vi "4155C Split array.vi"(0 "Number of VAR2 steps":i32, 1 "Y2 data in":dbl[](array[numeric]) format="%.2f", 2 "X data in":dbl[](array[numeric]) format="%.2f", 3 "Y1 data in":dbl[](array[numeric]) format="%.2f", 4 "Y3 data in":dbl[](array[numeric]) format="%.2f", 5 "error in (no error)":errorcluster, 8 "Absolute val?":bool=TRUE) -> (6 "Array of clusters":cluster{"Y data in":dbl[], "X data in":dbl[]}[](array[cluster]) {"X data in" format="%.2f"; "Y data in" format="%.2f"}, 7 "error out":errorcluster)   [LabVIEW 2019]
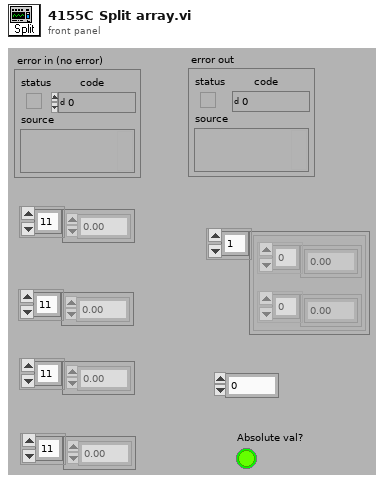
[diagram p1: front panel]
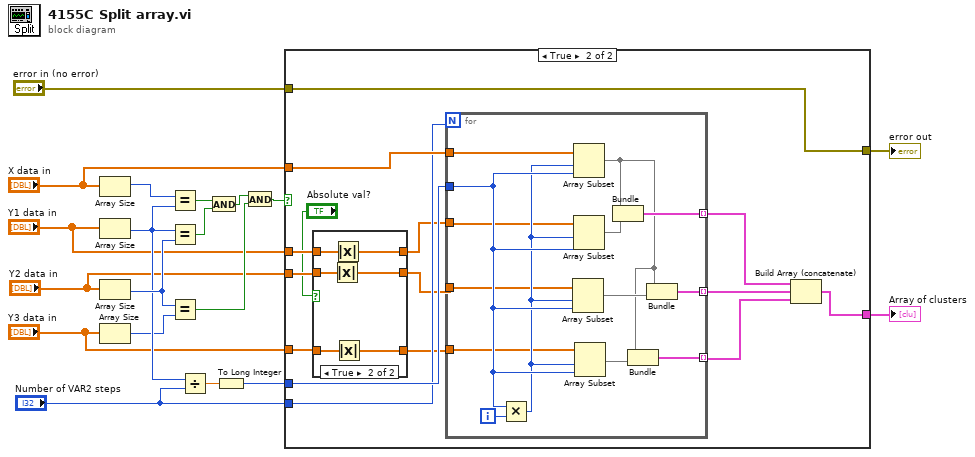
[diagram p0: block diagram]
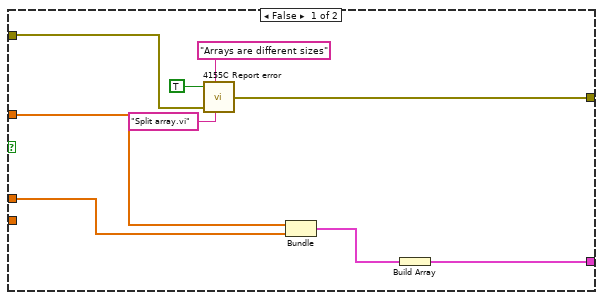
[diagram p2: hidden frame]
diagram:
  n1 = Array Size(array="X data in") -> (size(s)=w19:i32)
  n2 = Array Size(array="Y1 data in") -> (size(s)=w11:i32)
  n3 = Array Size(array="Y2 data in") -> (size(s)=w12:i32)
  n4 = Array Size(array="Y3 data in") -> (size(s)=w5:i32)
  n5 = Equal?(x=w19, y=w11) -> (x = y?=w10:bool)
  n6 = Equal?(x=w11, y=w12) -> (x = y?=w9:bool)
  n7 = Equal?(x=w12, y=w5) -> (x = y?=w6:bool)
  n8 = Divide(x=w11, y="Number of VAR2 steps") -> (x/y=w14:dbl)
  n9 = And(x=w10, y=w9) -> (x .and. y?=w7:bool)
  n10 = To Long Integer(number=w14) -> (32bit integer=w13:i32)
  n11 = And(x=w7, y=w6) -> (x .and. y?=w8:bool)
  n12 = case shown="True" w8 {
    tunnel: "X data in" -> [w23 w42]
    tunnel: "Y1 data in" -> [w22 w35]
    tunnel: "error in (no error)" -> [w28 w43]
    tunnel: [w27 w43] -> w17
    tunnel: "Number of VAR2 steps" -> [_ w40]
    tunnel: [w20 w39] -> w16
    tunnel: w13 -> [_ w41]
    tunnel: "Y2 data in" -> [_ w34]
    tunnel: "Y3 data in" -> [_ w32]
    frame False {
      n13 = call "4155C Report error.vi"("new error"=TRUE, "error message"="Arrays are different sizes", "error in (no error)"=w28, "source"="Split array.vi") -> ("error out"=w27:errorcluster)  [unwired: 1 in]
      n14 = Bundle("X data in"=w23, "Y1 data in"=w22) -> (w21:cluster{"X data in":dbl[], "Y1 data in":dbl[]})  [unwired: 1 in]
      n15 = Build Array(w21) -> (w20:cluster{"X data in":dbl[], "Y1 data in":dbl[]}[])
    }
    frame True {
      n16 = case shown="True" "Absolute val?" {
        tunnel: w35 -> [w44 w52]
        tunnel: [w46 w48] -> w33
        tunnel: w34 -> [w46 w51]
        tunnel: w32 -> [w45 w50]
        tunnel: [w45 w47] -> w31
        tunnel: [w44 w49] -> w29
        frame False {
        }
        frame True {
          n17 = Absolute Value(x=w51) -> (abs(x)=w48:dbl[])
          n18 = Absolute Value(x=w52) -> (abs(x)=w49:dbl[])
          n19 = Absolute Value(x=w50) -> (abs(x)=w47:dbl[])
        }
      }
      n20 = for {
        N: w40 -> [_]
        tunnel: w29 -> [w53]
        tunnel: w42 -> [w65]
        tunnel: [w66] -> w36 mode=indexing
        tunnel: w41 -> [w62]
        tunnel: w33 -> [w60]
        tunnel: w31 -> [w59]
        tunnel: [w55] -> w37 mode=indexing
        tunnel: [w54] -> w38 mode=indexing
        i -> [w64]
        n21 = Multiply(x=w62, y=w64) -> (x*y=w61:i32)
        n22 = Array Subset(array=w60, index=w61, length=w62) -> (w58:dbl[])
        n23 = Array Subset(array=w65, index=w61, length=w62) -> (w56:dbl[])
        n24 = Array Subset(array=w53, index=w61, length=w62) -> (w63:dbl[])
        n25 = Array Subset(array=w59, index=w61, length=w62) -> (w57:dbl[])
        n26 = Bundle(w56, w63) -> (w66:cluster{dbl[], dbl[]})  [unwired: 1 in]
        n27 = Bundle(w56, w57) -> (w54:cluster{dbl[], dbl[]})  [unwired: 1 in]
        n28 = Bundle(w56, w58) -> (w55:cluster{dbl[], dbl[]})  [unwired: 1 in]
      }
      n29 = Build Array (concatenate)(w36, w37, w38) -> (w39:cluster{dbl[], dbl[]}[])
    }
  }
  "error out" <- w17
  "Array of clusters" <- w16
